vi "MT Generate Bits (Fibonacci, PN Order).vi"(0 "total bits (128)":i32=128, 7 "PN sequence order":i32=9, 9 "seed in (0xD6BF7DF2)":i32=169 format="%.0b", 11 "error in (no error)":errorcluster, 13 "reset? (T)":bool=TRUE) -> (4 "output bit stream":i8[](array[numeric]), 10 "seed out":i32 format="%.0x", 15 "error out":errorcluster)   [LabVIEW 2020, in "niDMT.lvlib"]
doc: "This polymorphic instance generates Fibonacci pseudonoise (PN) bit sequences. The VI repeats the selected pattern until it generates the number of bits that you specify. Use this instance to specify a PN sequence order based on which the VI selects a primitive polynomial that returns an m-sequence."
uses:
  <vilib>/addons/Modulation/niDMT.lvlib
  <vilib>/addons/Modulation/Digital/Support/Common/mod_Number to Bits.vi
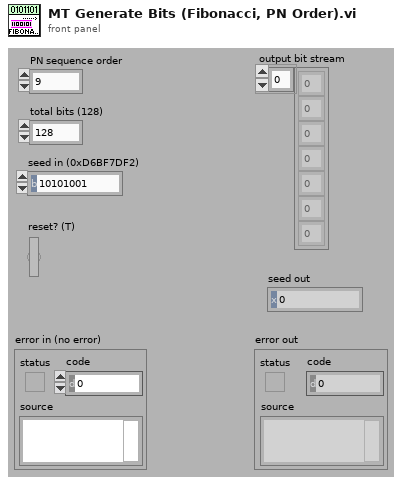
[diagram p1: front panel]
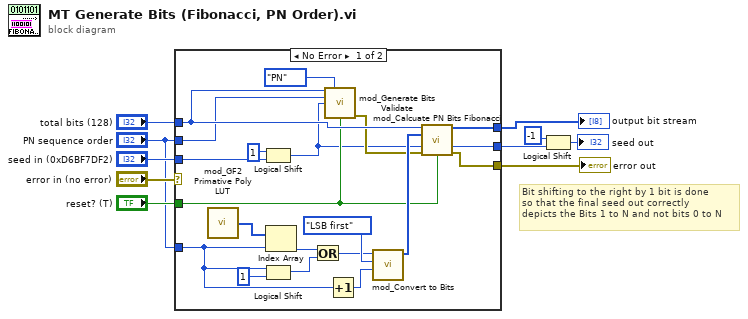
[diagram p0: block diagram]
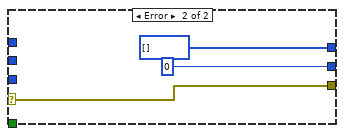
[diagram p2: hidden frame]
diagram:
  # "Bit shifting to the right by 1 bit is done \nso that the final seed out correctly \ndepicts the Bits 1 to N and not bits 0 to N"
  n1 = case shown="No Error" "error in (no error)" {
    selector: "error in (no error)" -> [_ w31]
    tunnel: "seed in (0xD6BF7DF2)" -> [w12 _]
    tunnel: "total bits (128)" -> [w18 _]
    tunnel: "PN sequence order" -> [w17 _]
    tunnel: [w19 i8[] []] -> w8
    tunnel: [w21 w31] -> w6
    tunnel: [w20 0] -> w1
    tunnel: "reset? (T)" -> [w15 _]
    tunnel: "PN sequence order" -> [w23 _]
    frame No Error {
      n2 = call <vilib>:"mod_GF2 Primative Poly LUT.vi"() -> ("GF(2) Primative Polynomials"=w24:u32[])
      n3 = Logical Shift(y=1, x=w12) -> (x << y=w11:i32)
      n4 = Logical Shift(y=w23, x=u32 1) -> (x << y=w26:u32)
      n5 = Index Array(array=w24, index=w23) -> (element=w27:u32)
      n6 = Or(x=w27, y=w26) -> (x .or. y?=w28:u32)
      n7 = call <vilib>:"mod_Generate Bits Validate.vi"("Total Bits"=w18, "Mode (PN)"=enum16{"PN", "pattern", "user"}."PN", "PN Sequence Order"=w17, "seed in"=w11, "reset?"=w15) -> ("error out"=w14:errorcluster)  [unwired: 2 in, 8 out]
      n8 = Increment(x=w23) -> (x+1=w30:i32)
      n9 = call-poly <vilib>:"mod_Convert to Bits.vi"("number of bits"=w30, "bit order"=enum16{"MSB first", "LSB first"}."LSB first", "Number"=w28) -> ("bits"=w22:i8[])  [unwired: 8 out]
      n10 = call <vilib>:"mod_Calcuate PN Bits Fibonacci.vi"("total bits (128)"=w18, "primitive polynomial"=w22, "seed in (0xD6BF7DF2)"=w11, "error in (no error)"=w14, "reset? (T)"=w15) -> ("output bits"=w19:i8[], "seed out"=w20:i32, "error out"=w21:errorcluster)  [unwired: 8 out]
    }
    frame Error {
    }
  }
  "output bit stream" <- w8
  "error out" <- w6
  n11 = Logical Shift(y=-1, x=w1) -> (x << y=→"seed out":i32)
